vi "Item with Settings to Tree Items.vi"(7 "item type":T1=enum."Group", 8 "error in (no error)":errorcluster, 9 "item index":i32, 10 "item name":string, 11 "Application Data in":T3) -> (0 "error out":errorcluster, 1 "Settings Item":T2, 2 "Item":T2, 3 "Application Data out":T3)   [LabVIEW 2019, in "DSF Configuration Utility.lvlib"]
uses:
  DSF Configuration Utility.lvlib
  Main VI/Application Data.ctl
  VeriStand/Data Sharing Custom Device/Source/DSF Core.lvlibp/Classes/Configuration Session/Configuration Session.lvclass
  Main VI/View Mode.ctl
  Tree Item.ctl
  Tree Item Type.ctl
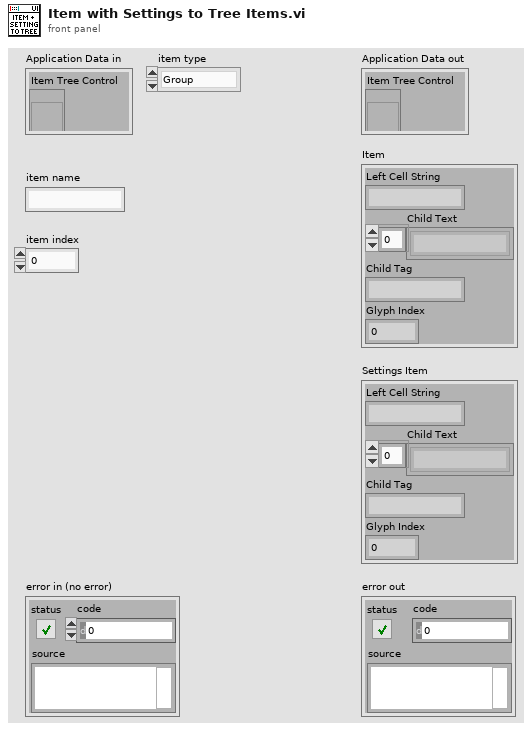
[diagram p1: front panel]
types:
  T1 = typedef "DSF Configuration Utility.lvlib/Tree Item Type.ctl" = enum16{"Plugin", "Group", "Transfer", "Channel", "Setting"}
  T2 = typedef "DSF Configuration Utility.lvlib/Tree Item.ctl" = cluster{"Left Cell String":string, "Child Text":string[], "Child Tag":string, "Glyph Index":i32}
  T3 = typedef "DSF Configuration Utility.lvlib/Application Data.ctl" = cluster{"Item Tree Control":refnum<vi>, "Value Tree Control":refnum<vi>, "Configuration Session":refnum<class "Configuration Session.lvclass">, "Top-Level VI":refnum<vi>, "View State":T4, "menu reference":refnum<k9>}
  T4 = typedef "DSF Configuration Utility.lvlib/View Mode.ctl" = enum16{"Tree", "List"}
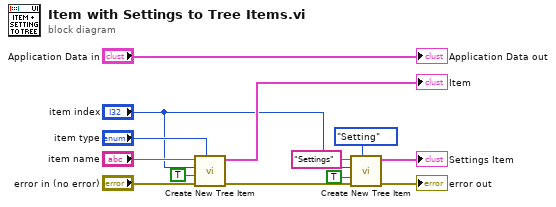
[diagram p0: block diagram]
diagram:
  n1 = call "Create New Tree Item.vi"("Item Type"="item type", "error in"="error in (no error)", "found?"=TRUE, "index"="item index", "Left Cell String"="item name") -> ("error out"=w6:errorcluster, "Item"=→"Item":T2)  [unwired: 5 in]
  n2 = call "Create New Tree Item.vi"("Item Type"=Tree_Item_Type."Setting", "error in"=w6, "found?"=TRUE, "index"="item index", "Left Cell String"="Settings") -> ("error out"=→"error out":errorcluster, "Item"=→"Settings Item":T2)  [unwired: 5 in]
  "Application Data out" <- "Application Data in"
